vi "Post Media Tweet - From File.vi"(8 "error in":errorcluster, 9 "Picture File (PNG, JPG, GIF)":path, 10 "Tweet":string, 11 "Twitter Handle In":T1={"OAuth Credentials"={"Signature Method"=enum."HMAC-SHA1", "Version"="1.0", "Client"={"Token"="", "Secret"=""}, "Access"={"Token"="", "Secret"=""}}, "since ID"="", "max ID"="", "Screen Name"=""}) -> (0 "error out":errorcluster, 3 "Twitter Handle Out":T1={"OAuth Credentials"={"Signature Method"=enum."HMAC-SHA1", "Version"="1.0", "Client"={"Token"="", "Secret"=""}, "Access"={"Token"="", "Secret"=""}}, "since ID"="", "max ID"="", "Screen Name"=""})   [LabVIEW 2011, in "i3-twitter.lvlib"]
doc: "Posts a status update as a Tweet for the authenticated user that includes a picture file in a supported format (.png, .jpg, .gif). Duplicate posts will result in an error message from Twitter."
uses:
  i3-twitter.lvlib
  Controls/Twitter Handle.ctl
  i3-oauth/Controls/OAuth Handle.ctl
  i3-oauth/Controls/Signature Method.ctl
  i3-oauth/Controls/Credentials.ctl
  <vilib>/httpClient/MultipartData.ctl
  i3-oauth/Controls/HTTP Method.ctl
  i3-oauth/i3-oauth.lvlib
  <vilib>/httpClient/LabVIEWHTTPClient.lvlib
panel:
  out "headers (response)":string
  out "body (response)":string
  out "Full URL":string
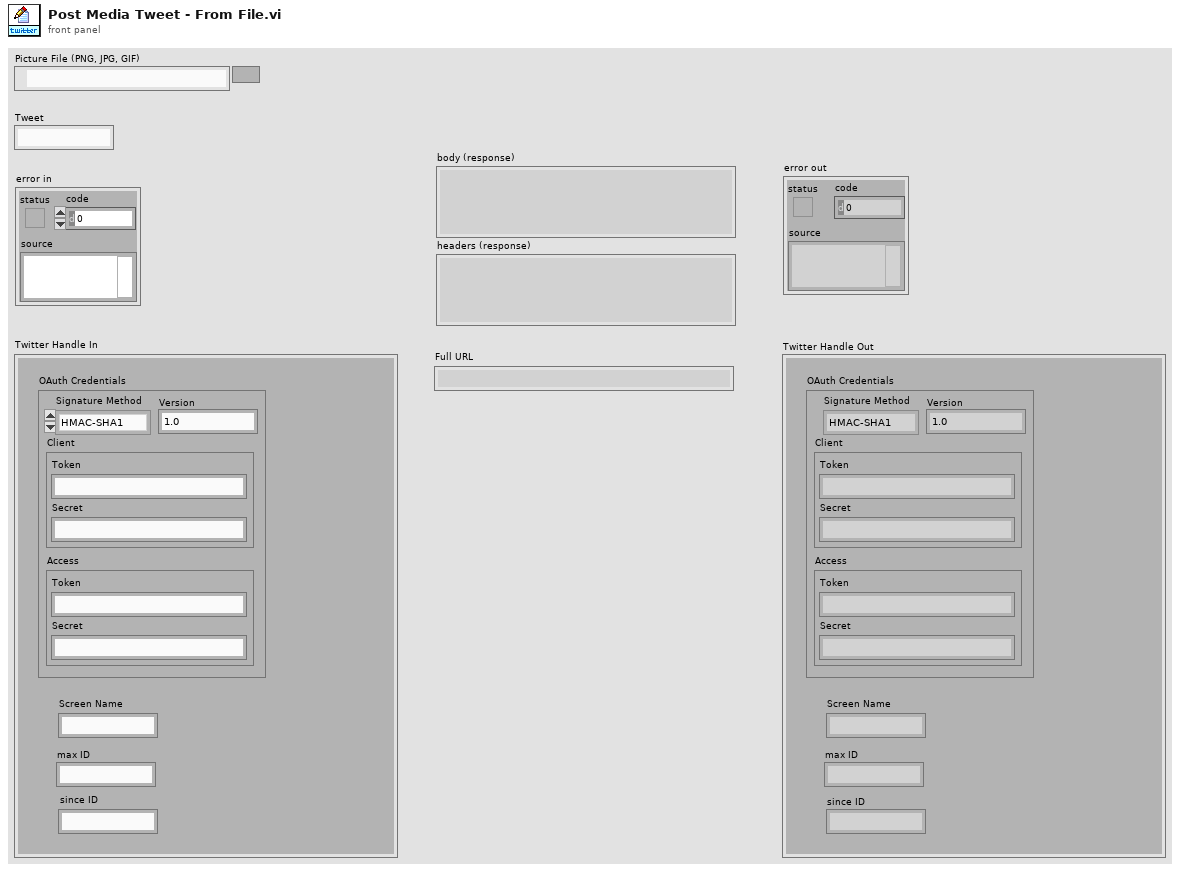
[diagram p1: front panel]
types:
  T1 = typedef "i3-twitter.lvlib/Twitter Handle.ctl" = cluster{"OAuth Credentials":T2, "since ID":string, "max ID":string, "Screen Name":string}
  T2 = typedef "i3-oauth.lvlib/OAuth Handle.ctl" = cluster{"Signature Method":T3, "Version":string, "Client":T4, "Access":T4}
  T3 = typedef "i3-oauth.lvlib/Signature Method.ctl" = enum16{"HMAC-MD5", "HMAC-SHA1", "HMAC-SHA224", "HMAC-SHA256", "HMAC-SHA384", "HMAC-SHA512"}
  T4 = typedef "i3-oauth.lvlib/Credentials.ctl" = cluster{"Token":string, "Secret":string}
  T5 = typedef "LabVIEWHTTPClient.lvlib/MultipartData.ctl" = cluster{"Name":string, "Value":string, "File":path, "Filename":string, "MIME type":string}
  T6 = typedef "i3-oauth.lvlib/HTTP Method.ctl" = enum16{"GET", "POST", "PUT", "DELETE"}
  T7 = typedef "LabVIEWHTTPClient.lvlib/ClientHandle.ctl" = refnum<k1>
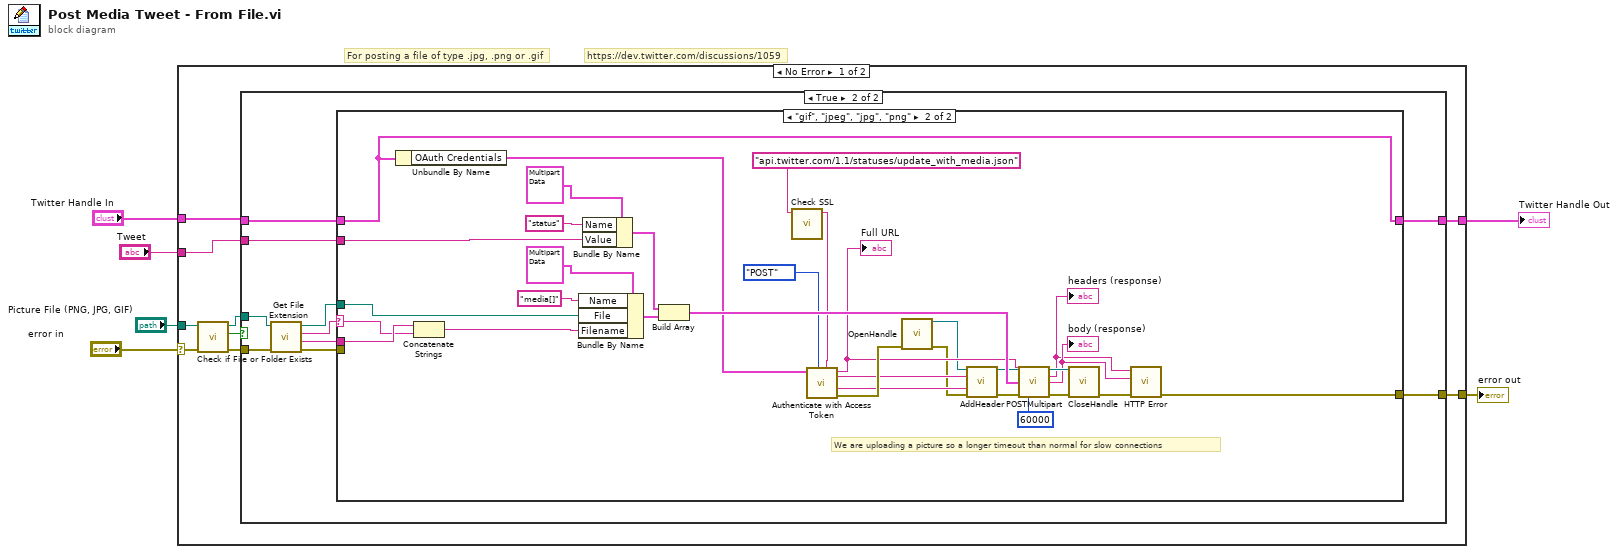
[diagram p0: block diagram]
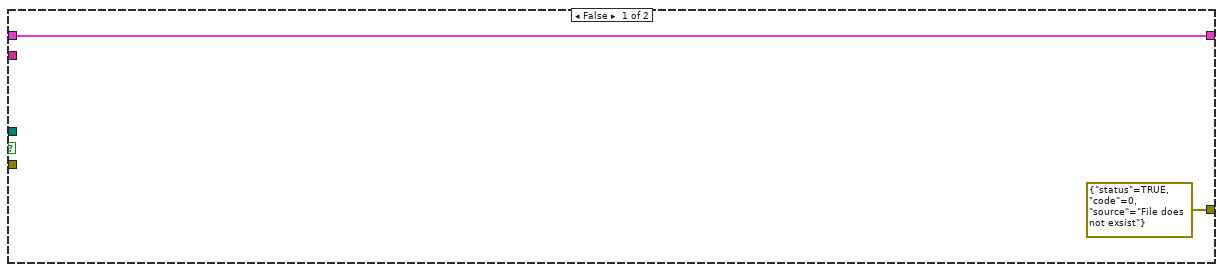
[diagram p2: hidden frame]
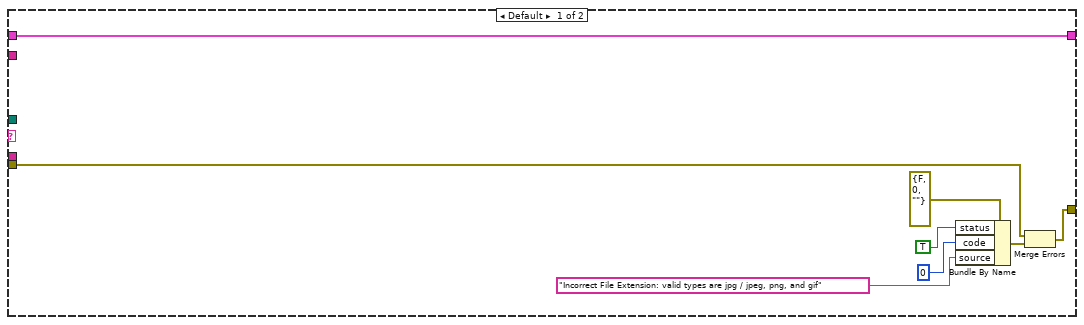
[diagram p3: hidden frame]
diagram:
  # "For posting a file of type .jpg, .png or .gif"
  # "https://dev.twitter.com/discussions/1059"
  n1 = case shown="No Error" "error in" {
    selector: "error in" -> [w7 w69]
    tunnel: [w15 w69] -> w5
    tunnel: "Picture File (PNG, JPG, GIF)" -> [w14 _]
    tunnel: "Twitter Handle In" -> [w11 w68]
    tunnel: "Tweet" -> [w10 _]
    tunnel: [w9 w68] -> w1
    frame No Error {
      n2 = call <vilib>:"Check if File or Folder Exists.vi"("error in (no error)"=w7, "path"=w14) -> ("error out"=w8:errorcluster, "file or folder exists?"=w13:bool, "dup path"=w12:path)  [unwired: 7 in]
      n3 = case shown="True" w13 {
        tunnel: [errorcluster {"status"=TRUE, "code"=0, "source"="File does not exsist"} ("error out") w27] -> w15
        tunnel: w12 -> [_ w26]
        tunnel: w11 -> [w16 w23]
        tunnel: w10 -> [_ w22]
        tunnel: [w16 w21] -> w9
        tunnel: w8 -> [_ w19]
        frame False {
        }
        frame True {
          n4 = call <vilib>:"Get File Extension.vi"("error in (no error)"=w19, "file"=w26) -> ("error out"=w18:errorcluster, "filename without extension"=w20:string, "lowercase file extension"=w25:string, "dup file"=w24:path)  [unwired: 6 in]
          n5 = case shown="\"gif\", \"jpeg\", \"jpg\", \"png\"" w25 {
            selector: w25 -> [_ w41]
            tunnel: [w29 w46] -> w27
            tunnel: w24 -> [_ w49]
            tunnel: w23 -> [w35 w43]
            tunnel: w22 -> [_ w48]
            tunnel: [w35 w43] -> w21
            tunnel: w20 -> [_ w42]
            tunnel: w18 -> [w28 _]
            frame Default {
              n6 = Bundle By Name(cluster=errorcluster {"status"=FALSE, "code"=0, "source"=""} ("error in (no error)"), "status"=TRUE, "code"=0, "source"="Incorrect File Extension: valid types are jpg / jpeg, png, and gif") -> (w30:errorcluster)
              n7 = Merge Errors(w28, w30) -> (w29:errorcluster)
            }
            frame "gif", "jpeg", "jpg", "png" {
              # "We are uploading a picture so a longer timeout than normal for slow connections"
              n8 = Unbundle By Name(w43) -> ("OAuth Credentials"=w39:T2)
              n9 = Concatenate Strings(w42, w41) -> (w50:string)
              n10 = Bundle By Name(cluster=T5 {"Name"="", "Value"="", "File"=path "", "Filename"="", "MIME type"="application/octet-stream"} ("Element"), "Name"="media[]", "File"=w49, "Filename"=w50) -> (w65:T5)
              n11 = Bundle By Name(cluster=T5 {"Name"="", "Value"="", "File"=path "", "Filename"="", "MIME type"="application/octet-stream"} ("Element"), "Name"="status", "Value"=w48) -> (w61:T5)
              n12 = Build Array(w61, w65) -> (w62:T5[])
              n13 = call "Check SSL.vi"("Input URL"="api.twitter.com/1.1/statuses/update_with_media.json" ("Base URL")) -> ("Output URL"=w38:string)  [unwired: 8 in]
              n14 = call "Authenticate with Access Token.vi"("Base URL"=w38, "HTTP Method"=HTTP_Method."POST", "OAuth Handle"=w39) -> ("error out"=w67:errorcluster, "Header Value"=w54:string, "Header Parameter"=w53:string, "Full URL"=w59:string)  [unwired: 4 in, 1 out]
              "Full URL" <- w59
              n15 = call <vilib>:"OpenHandle.vi"("error in (no error)"=w67) -> ("client handle out"=w51:T7, "error out"=w52:errorcluster)  [unwired: 13 in]
              n16 = call <vilib>:"AddHeader.vi"("client handle"=w51, "header"=w53, "value"=w54, "error in (no error)"=w52) -> ("client handle out"=w55:T7, "error out"=w56:errorcluster)  [unwired: 10 in]
              n17 = call <vilib>:"POSTMultipart.vi"("client handle"=w55, "url"=w59, "data"=w62, "error in (no error)"=w56, "timeout (10000)"=60000) -> ("client handle out"=w58:T7, "headers"=w44:string, "body"=w45:string, "error out"=w57:errorcluster)  [unwired: 7 in]
              "body (response)" <- w45
              "headers (response)" <- w44
              n18 = call <vilib>:"CloseHandle.vi"("client handle"=w58, "error in (no error)"=w57) -> ("error out"=w47:errorcluster)  [unwired: 13 in]
              n19 = call "HTTP Error.vi"("error in (no error)"=w47, "Body"=w45, "Header"=w44) -> ("error out"=w46:errorcluster)  [unwired: 6 in, 2 out]
            }
          }
        }
      }
    }
    frame Error {
    }
  }
  "error out" <- w5
  "Twitter Handle Out" <- w1
